vi "data_decimate.vi"   [LabVIEW 2017]
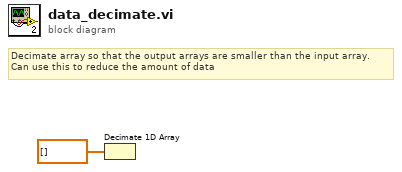
[diagram p0: block diagram]
diagram:
  # "Decimate array so that the output arrays are smaller than the input array.\nCan use this to reduce the amount of data"
  n1 = Decimate 1D Array(dbl[] [] ("array")) -> ()  [unwired: 2 out]
